vi "Read_AI.vi"(11 "VISA resource name":refnum<visa-resource-name>) -> (0 "VISA resource name out":refnum<visa-resource-name>, 3 "Numeric":dbl)   [LabVIEW 2016]
uses:
  <vilib>/Analysis/3filter.llb/Filter Passband Type.ctl
  <vilib>/ptbypt/NI_PtbyPt.lvlib
  <vilib>/Analysis/NI_AALBase.lvlib
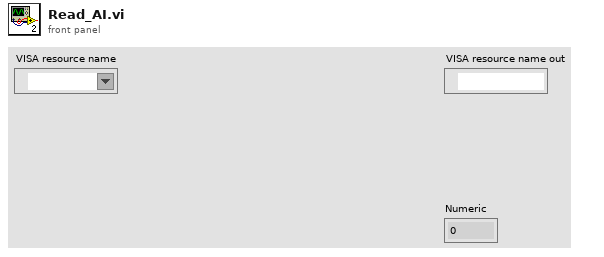
[diagram p1: front panel]
types:
  T1 = typedef "NI_AALBase.lvlib/Filter Passband Type.ctl" = enum32{"Lowpass", "Highpass", "Bandpass", "Bandstop"}
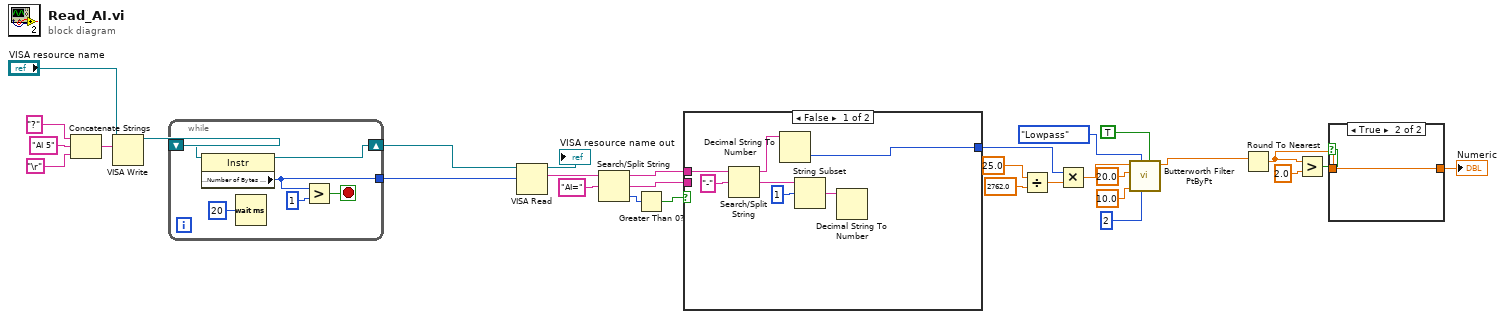
[diagram p0: block diagram]
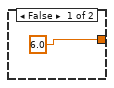
[diagram p2: hidden frame]
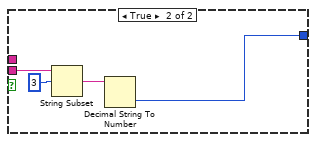
[diagram p3: hidden frame]
diagram:
  n1 = Concatenate Strings("?" ("string to write 2"), "AI 5" ("string"), "\r") -> (w18:string)
  n2 = VISA Write(VISA resource name="VISA resource name", write buffer=w18) -> (VISA resource name out=w16:refnum<visa-resource-name>)  [unwired: 1 in, 2 out]
  n3 = while {
    shift-right: [w35] -> w17
    shift-left: w16 -> [w36]
    tunnel: [w32] -> w27
    stop <- w33 stop-if-true
    n4 = property class="Instr"(reference=w36) -> (reference out=w35:refnum<visa-resource-name>, "Serial Settings:Number of Bytes at Serial Port"=w32:u32)  [unwired: 1 in, 1 out]
    n5 = Wait (ms)(milliseconds to wait=u32 20) -> ()  [unwired: 1 out]
    n6 = Greater?(x=w32, y=u32 1) -> (0:w33:bool)
  }
  n7 = VISA Read(VISA resource name=w17, byte count=w27) -> (VISA resource name out=→"VISA resource name out":refnum<visa-resource-name>, read buffer=w26:string)  [unwired: 1 in, 2 out]
  n8 = Search/Split String(string=w26, search string/char (-)="AI=") -> (substring before match=w25:string, match + rest of string=w22:string, offset of match=w23:i32)  [unwired: 1 in]
  n9 = Greater Than 0?(x=w23) -> (x > 0?=w24:bool)
  n10 = case shown="False" w24 {
    tunnel: [w40 w44] -> w5
    tunnel: w22 -> [_ w46]
    tunnel: w25 -> [w42 _]
    frame False {
      n11 = Search/Split String(string=w42, search string/char (-)="-") -> (substring before match=w41:string, match + rest of string=w39:string)  [unwired: 1 in, 1 out]
      n12 = Decimal String To Number(string=w41) -> (number=w40:i32)  [unwired: 2 in, 1 out]
      n13 = String Subset(string=w39, offset (0)=1) -> (substring=w37:string)  [unwired: 1 in]
      n14 = Decimal String To Number(string=w37) -> ()  [unwired: 2 in, 2 out]
    }
    frame True {
      n15 = String Subset(string=w46, offset (0)=3) -> (substring=w45:string)  [unwired: 1 in]
      n16 = Decimal String To Number(string=w45) -> (number=w44:i32)  [unwired: 2 in, 1 out]
    }
  }
  n17 = Divide(x=25.0, y=2762.0) -> (x/y=w6:dbl)
  n18 = Multiply(x=w5, y=w6) -> (x*y=w14:dbl)
  n19 = call <vilib>:"Butterworth Filter PtByPt.vi"("initialize"=TRUE, "order"=2, "filter type"=Filter_Passband_Type."Lowpass", "low cutoff freq: fl"=10.0, "sampling freq: fs"=20.0, "x"=w14) -> ("Filtered x"=w1:dbl)  [unwired: 3 in, 1 out]
  n20 = Round To Nearest(number=w1) -> (nearest integer value=w30:dbl)
  n21 = Greater?(x=w30, y=2.0) -> (0:w29:bool)
  n22 = case shown="True" w29 {
    tunnel: w30 -> [_ w49]
    tunnel: [6.0 w49] -> w4
    frame False {
    }
    frame True {
    }
  }
  "Numeric" <- w4
